vi "Test ARGB to-from Greyscale.vi"(8 "error in (no error)":errorcluster, 11 "Test Case In":refnum<class "Image.lvclass">) -> (0 "error out":errorcluster, 3 "Test Case Out":refnum<class "Image.lvclass">)   [LabVIEW 2020, in "g_ar_toolkit.test.lvlib" / "Image.lvclass"]
uses:
  Image.lvclass
  C:/Program Files (x86)/National Instruments/LabVIEW 2020/vi.lib/Astemes/LUnit/Test Case.lvclass
  g_ar_toolkit.common/Image Size (Integer).ctl
  <vilib>/Astemes/LUnit/Test Case.lvclass/Test Case.ctl
  g_ar_toolkit.image/CreateEmptyImageGreyscale.vi
  g_ar_toolkit.image/CreateEmptyImageARGB.vi
  4993e8ee-a06a-463a-9684-69129f64d5ce.vi
  g_ar_toolkit.image/Copy Array to Image.vi
  g_ar_toolkit.image/CopyArrayToImageARGB.vi
  g_ar_toolkit.image/CreateEmptyImageGreyscale.vi/6598b9e0-8a08-46f5-91fd-ca1b87217137.vi
  g_ar_toolkit.image/ARGBExtractChannel.vi
  g_ar_toolkit.image/CreateEmptyImageARGB.vi/3321fa97-f432-4e1e-8db9-a0df79aed21b.vi
  <vilib>/Astemes/LUnit/Append Pass Result.vi
  <vilib>/Astemes/LUnit/Append Fail Result.vi
  <vilib>/Astemes/LUnit/Describe Comparison.vi
  <vilib>/Astemes/LUnit/Compare Variants.vi
  g_ar_toolkit.image/CopyArrayToImageARGB.vi/26c70cee-9332-41f4-9755-08948a885cbe.vi
  <vilib>/Astemes/LUnit/Run In UI.vi
  <vilib>/Utility/error.llb/Clear Errors.vi
  g_ar_toolkit.image/ARGBColourToU32.vi
  g_ar_toolkit.common/Module Path.vi
  <vilib>/Utility/error.llb/Error Cluster From Error Code.vi
  <vilib>/picture/pixmap.llb/Flatten Pixmap.vi
  <vilib>/Astemes/LUnit/Describe Variant.vi
  Image.lvclass/Image.ctl
  g_ar_toolkit.image/g_ar_toolkit.image.lvlib
  g_ar_toolkit.common/g_ar_toolkit.common.lvlib
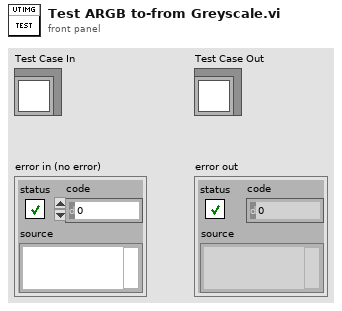
[diagram p1: front panel]
types:
  T1 = typedef "g_ar_toolkit.common.lvlib/Image Size (Integer).ctl" = cluster{"Width":u16, "Height":u16}
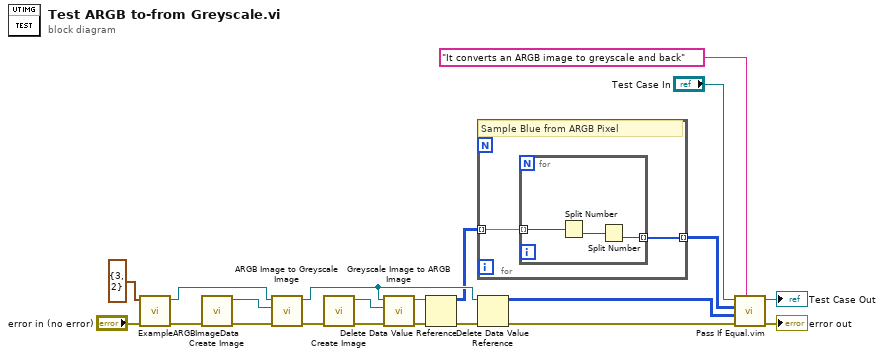
[diagram p0: block diagram]
diagram:
  n1 = call "ExampleARGBImageData.vi"("error in (no error)"="error in (no error)", "Image Size"=T1 {"Width"=3, "Height"=2}) -> ("error out"=w16:errorcluster, "Data Value Reference out"=w8:refnum<data-value>)  [unwired: 6 in, 2 out]
  n2 = call-poly "Create Image.vi"("error in (no error)"=w16) -> ("error out"=w14:errorcluster, "New Greyscale Image"=w17:refnum<data-value>)  [unwired: 9 in]
  n3 = call "ARGB Image to Greyscale Image.vi"("error in (no error)"=w14, "Greyscale Image Destination"=w17, "ARGB Image Source"=w8) -> ("error out"=w13:errorcluster, "Greyscale Image Destination (Duplicate)"=w7:refnum<data-value>)  [unwired: 7 in]
  n4 = call-poly "Create Image.vi"("error in (no error)"=w13) -> ("error out"=w11:errorcluster, "New ARGB Image"=w12:refnum<data-value>)  [unwired: 9 in]
  n5 = call "Greyscale Image to ARGB Image.vi"("error in (no error)"=w11, "ARGB Image Destination"=w12, "Greyscale Image Source"=w7) -> ("error out"=w9:errorcluster, "ARGB Image Destination (Duplicate)"=w10:refnum<data-value>)  [unwired: 7 in]
  n6 = Delete Data Value Reference(data value reference=w10, error in=w9) -> (data value=w3:u32[][], error out=w6:errorcluster)
  n7 = for {
    tunnel: w3 -> [w23] mode=indexing
    tunnel: [w22] -> w2 mode=indexing
    # "Sample Blue from ARGB Pixel"
    n8 = for {
      tunnel: w23 -> [w26] mode=indexing
      tunnel: [w24] -> w22 mode=indexing
      n9 = Split Number(x=w26) -> (lo(x)=w25:u16)  [unwired: 1 out]
      n10 = Split Number(x=w25) -> (lo(x)=w24:u8)  [unwired: 1 out]
    }
  }
  n11 = Delete Data Value Reference(data value reference=w7, error in=w6) -> (data value=w4:u8[][], error out=w5:errorcluster)
  n12 = call "Pass If Equal.vim"("Description"="It converts an ARGB image to greyscale and back", "error in (no error)"=w5, "Actual"=w4, "Expected"=w2, "LUnit Test Case In"="Test Case In") -> ("error out"=→"error out":errorcluster, "LUnit Test Case Out"=→"Test Case Out":refnum<class "Image.lvclass">)  [unwired: 5 in]
